vi "Filter LLB Files.vi"(1 "Generated Files in":string[](array[string]), 2 "Filter Array":string[](array[string])=["Configuration", "_depinstr.bin", ".llb", "Windows"]) -> (0 "Generated Files out":string[](array[string]))   [LabVIEW 2019, in "Project XML Editor.lvclass"]
uses:
  Project XML Editor.lvclass
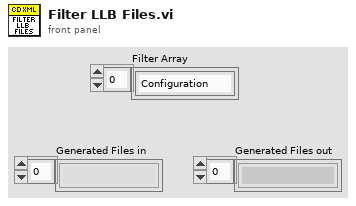
[diagram p1: front panel]
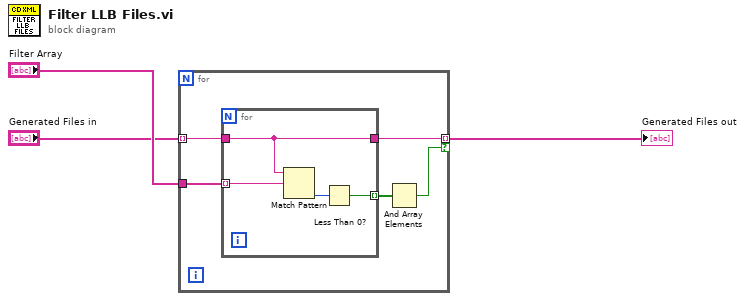
[diagram p0: block diagram]
diagram:
  n1 = for {
    tunnel: "Generated Files in" -> [w7] mode=indexing
    tunnel: "Filter Array" -> [w6]
    tunnel: [w5] -> w3 mode=indexing if=w4
    n2 = for {
      tunnel: w7 -> [w10]
      tunnel: w6 -> [w12] mode=indexing
      tunnel: [w10] -> w5
      tunnel: [w9] -> w8 mode=indexing
      n3 = Match Pattern(string=w10, regular expression=w12) -> (offset past match=w11:i32)  [unwired: 1 in, 3 out]
      n4 = Less Than 0?(x=w11) -> (x < 0?=w9:bool)
    }
    n5 = And Array Elements(Boolean array=w8) -> (logical AND=w4:bool)
  }
  "Generated Files out" <- w3
